vi "prepare function list.vi"(5 "sort?":bool, 6 "error in":errorcluster, 8 "Functions listbox":refnum<vi>, 9 "configuration in":refnum<class "user tag bus module configuration.lvclass">) -> (0 "error out":errorcluster)   [LabVIEW 2013, in "user tag bus module editor node.lvclass"]
uses:
  user tag bus module editor node.lvclass
  module/configuration/user tag bus module configuration.lvclass
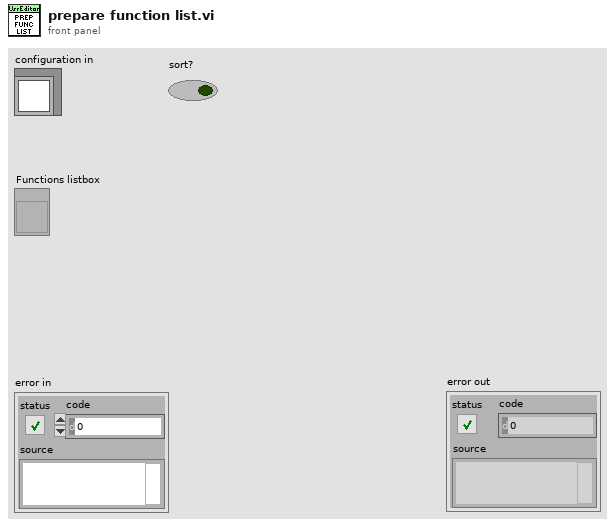
[diagram p1: front panel]
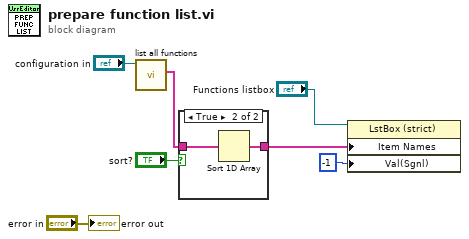
[diagram p0: block diagram]
diagram:
  n1 = call "list all functions.vi"("user module configuration in"="configuration in") -> ("functions"=w2:string[])  [unwired: 9 in, 1 out]
  n2 = case shown="True" "sort?" {
    tunnel: [w8 w9] -> w3
    tunnel: w2 -> [w8 w10]
    frame False {
    }
    frame True {
      n3 = Sort 1D Array(array=w10) -> (sorted array=w9:string[])
    }
  }
  n4 = property class="LstBox (strict)"(reference="Functions listbox", "Item Names"=w3, "Val(Sgnl)"=-1 ("Value (Signaling)")) -> ()  [unwired: 1 in, 2 out]
  "error out" <- "error in"
